vi "Intan_Sampling_and_MaxStreamChans.vi"(0 "VISA resource name":refnum<visa-resource-name>="COM1", 1 "error in":errorcluster, 2 "Desired Fs (Hz)":u16=100) -> (4 "VISA resource name out":refnum<visa-resource-name>, 5 "error out":errorcluster, 6 "NstreamChansmax":i32, 7 "FS actual (Hz)":i32, 8 "Actual Sampling Frequency (Hz)":string, 9 "NchansmaxStr":string)   [LabVIEW 2017]
doc: "use this VI to set the sampling rate (number samples/s/channel). Specify the rate in Hz. \nThis VI also computes the maximum number of channels that can be streameda the sampling rate. \nIn effect, this sets the intervalTimer object on the Teensyduino to precisely time ADC conversions. \nConversion time for 32 channels occurs in tens of microseconds typically."
panel:
  out "Max Chans Streamed at Fs":string
  out "ack string":string
  out "Teensy fs string written (Fs desired)":string
  in  "Teensy event char":string="m"
  # "ADC Sampilng"
  # "Max Chans Streaming"
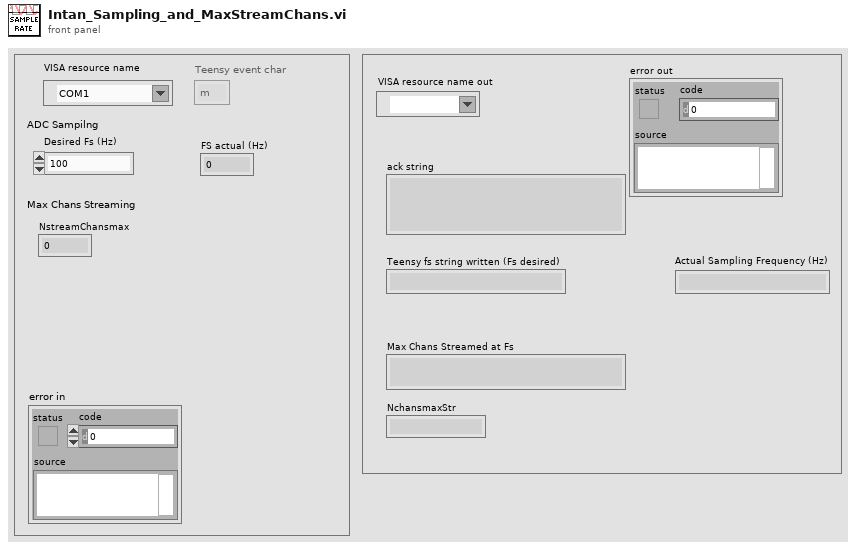
[diagram p1: front panel]
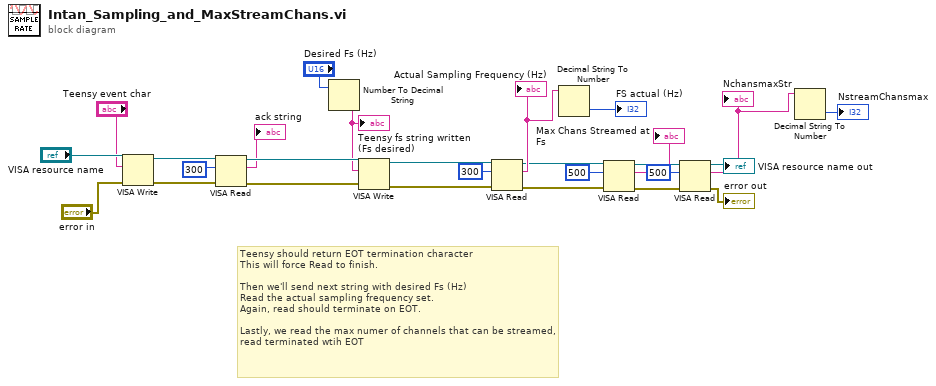
[diagram p0: block diagram]
diagram:
  # "Teensy should return EOT termination character \nThis will force Read to finish.\n\nThen we'll send next string with desired Fs (Hz)\nRead the actual sampling frequency set.\nAgain, read should terminate on EOT.\n\nLastly, we read the max numer of channels that can be streamed,\nread terminated wtih EOT"
  n1 = VISA Write(VISA resource name="VISA resource name", write buffer="Teensy event char", error in (no error)="error in") -> (VISA resource name out=w19:refnum<visa-resource-name>, error out=w18:errorcluster)  [unwired: 1 out]
  n2 = VISA Read(VISA resource name=w19, byte count=u32 300, error in (no error)=w18) -> (VISA resource name out=w25:refnum<visa-resource-name>, read buffer=→"ack string":string, error out=w24:errorcluster)  [unwired: 1 out]
  n3 = Number To Decimal String(number="Desired Fs (Hz)") -> (decimal integer string=w21:string)  [unwired: 1 in]
  "Teensy fs string written (Fs desired)" <- w21
  n4 = VISA Write(VISA resource name=w25, write buffer=w21, error in (no error)=w24) -> (VISA resource name out=w16:refnum<visa-resource-name>, error out=w15:errorcluster)  [unwired: 1 out]
  n5 = VISA Read(VISA resource name=w16, byte count=u32 300, error in (no error)=w15) -> (VISA resource name out=w11:refnum<visa-resource-name>, read buffer=w20:string, error out=w12:errorcluster)  [unwired: 1 out]
  "Actual Sampling Frequency (Hz)" <- w20
  n6 = Decimal String To Number(string=w20) -> (number=→"FS actual (Hz)":i32)  [unwired: 2 in, 1 out]
  n7 = VISA Read(VISA resource name=w11, byte count=u32 500, error in (no error)=w12) -> (VISA resource name out=w7:refnum<visa-resource-name>, read buffer=→"Max Chans Streamed at Fs":string, error out=w6:errorcluster)  [unwired: 1 out]
  n8 = VISA Read(VISA resource name=w7, byte count=u32 500, error in (no error)=w6) -> (VISA resource name out=→"VISA resource name out":refnum<visa-resource-name>, read buffer=w2:string, error out=→"error out":errorcluster)  [unwired: 1 out]
  "NchansmaxStr" <- w2
  n9 = Decimal String To Number(string=w2) -> (number=→"NstreamChansmax":i32)  [unwired: 2 in, 1 out]
